vi "LM 2D Gaussian + Flow ACF and gradient.vi"(3 "output control":T1, 4 "data":variant, 5 "X":dbl[](array[numeric]), 6 "a":dbl[](array[numeric])) -> (0 "error out":errorcluster, 1 "f'(X,a)":dbl[][](array[numeric]), 2 "f(X,a)":dbl[](array[numeric]))   [LabVIEW 2021, in "Fits.lvlib"]
doc: "This template is the starting point for creating a model function to be passed to the Nonlinear Curve Fit.vi."
uses:
  <vilib>/gmath/NumericalOptimization/LM_output select.ctl
  Fits.lvlib
  <vilib>/gmath/NI_Gmath.lvlib
panel:
  # "Parameters:\n\namplitude: A\ndiffusion time: tD\nTranslation time constant: tF"
  # "ACF(x) = 1 + A/(1 + x/tD)*exp(-(x/tF)^2/(1+x/tD))"
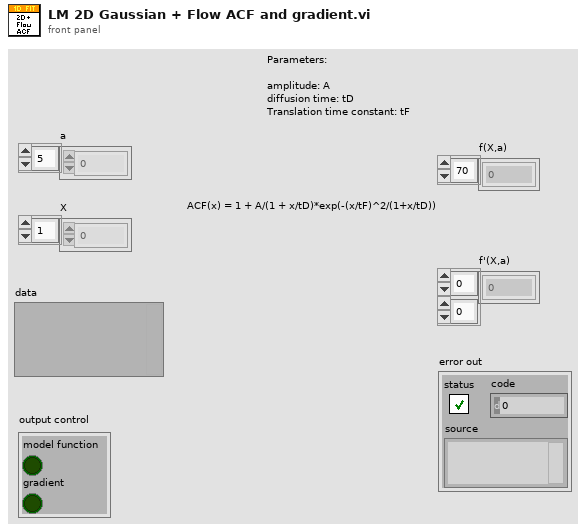
[diagram p1: front panel]
types:
  T1 = typedef "NI_Gmath.lvlib/LM_output select.ctl" = cluster{"model function":bool, "gradient":bool}
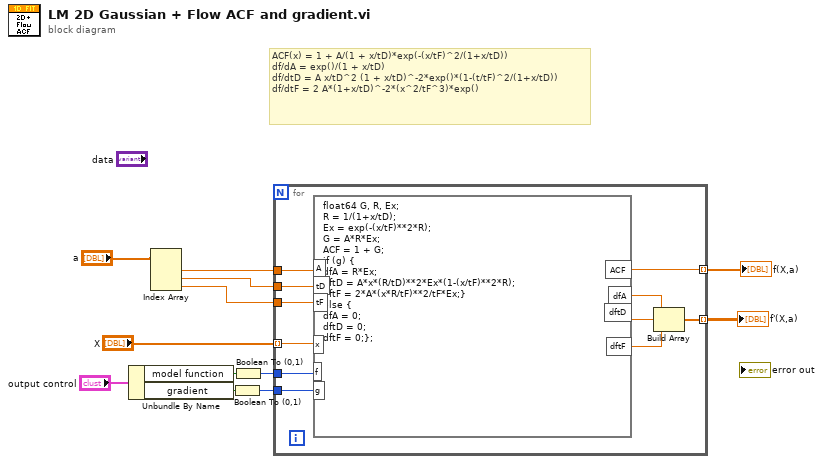
[diagram p0: block diagram]
diagram:
  # "ACF(x) = 1 + A/(1 + x/tD)*exp(-(x/tF)^2/(1+x/tD))\ndf/dA = exp()/(1 + x/tD)\ndf/dtD = A x/tD^2 (1 + x/tD)^-2*exp()*(1-(t/tF)^2/(1+x/tD))\ndf/dtF = 2 A*(1+x/tD)^-2*(x^2/tF^3)*exp()"
  n1 = Unbundle By Name("output control") -> ("model function"=w5:bool, "gradient"=w4:bool)
  n2 = Index Array(array="a") -> (element #1=w8:dbl, element #2=w7:dbl, element #3=w6:dbl)  [unwired: 3 in]
  n3 = Boolean To (0,1)(Boolean=w4) -> (0, 1=w1:i16)
  n4 = Boolean To (0,1)(Boolean=w5) -> (0, 1=w2:i16)
  n5 = for {
    tunnel: w8 -> [w22]
    tunnel: w7 -> [w23]
    tunnel: "X" -> [w21] mode=indexing
    tunnel: [w20] -> w10 mode=indexing
    tunnel: [w17] -> w9 mode=indexing
    tunnel: w6 -> [w16]
    tunnel: w2 -> [w14]
    tunnel: w1 -> [w13]
    n6 = formula code="float64 G, R, Ex;\nR = 1/(1+x/tD);\nEx = exp(-(x/tF)**2*R);\nG = A*R*Ex;\nACF = 1 + G;\nif (g) {\ndfA = R*Ex;\ndftD = A*x*(R/tD)**2*Ex*(1-(x/tF)**2*R);\ndftF = 2*A*(x*R/tF)**2/tF*Ex;}\nelse {\ndfA = 0;\ndftD = 0;\ndftF = 0;};"("A"=w22, "tD"=w23, "x"=w21, "tF"=w16, "f"=w14, "g"=w13) -> ("ACF"=w20:dbl, "dfA"=w19:dbl, "dftD"=w18:dbl, "dftF"=w15:dbl)
    n7 = Build Array(w19, w18, w15) -> (w17:dbl[])
  }
  "f(X,a)" <- w10
  "f'(X,a)" <- w9
